vi "HexToDword.vi"(11 "数组":u16[](array[numeric]) format="%04xH") -> (3 "DWORD":i32[](array[numeric]))   [LabVIEW 2016, in "挥发酚.lvlib"]
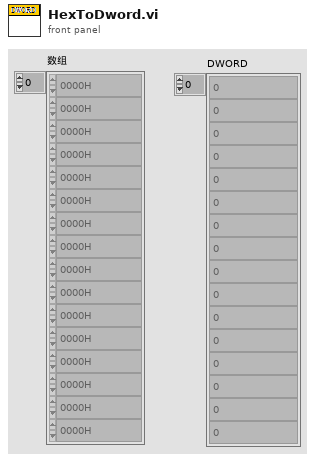
[diagram p1: front panel]
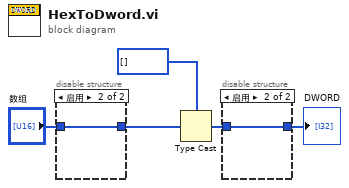
[diagram p0: block diagram]
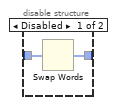
[diagram p2: hidden frame]
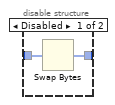
[diagram p3: hidden frame]
diagram:
  n1 = disable-structure shown="启用" {
    disable-tunnel: "数组" -> [w7 w8]
    disable-tunnel: [w6 w8] -> w4
    frame Disabled {
      n2 = Swap Bytes(anything=w7) -> (byte swapped=w6:u16[])
    }
    frame Enabled {
    }
  }
  n3 = Type Cast(type=i32[] [], x=w4) -> (*(type *) &x=w2:i32[])
  n4 = disable-structure shown="启用" {
    disable-tunnel: w2 -> [w10 w11]
    disable-tunnel: [w9 w11] -> w1
    frame Disabled {
      n5 = Swap Words(1:w10) -> (0:w9:i32[])
    }
    frame Enabled {
    }
  }
  "DWORD" <- w1
